vi "Remove Constant Current.vi"(0 "Device Name":string="Dev4", 1 "Device/Ports/Lines":string="Dev1/port0/line1,Dev1/port0/line5,Dev1/port0/line13,Dev1/port0/line15,Dev1/port0/line31,Dev1/port0/line30,Dev1/port0/line29,Dev1/port0/line26,Dev1/port0/line25,Dev1/port0/line24,Dev1/port0/line23,Dev1/port0/line22,Dev1/port0/line21,Dev1/port0/line20,Dev1/port0/line19,Dev1/port0/line18,Dev1/port0/line17\n", 3 "error in":errorcluster) -> (10 "error out":errorcluster)   [LabVIEW 2015]
panel:
  # "True means close relay"
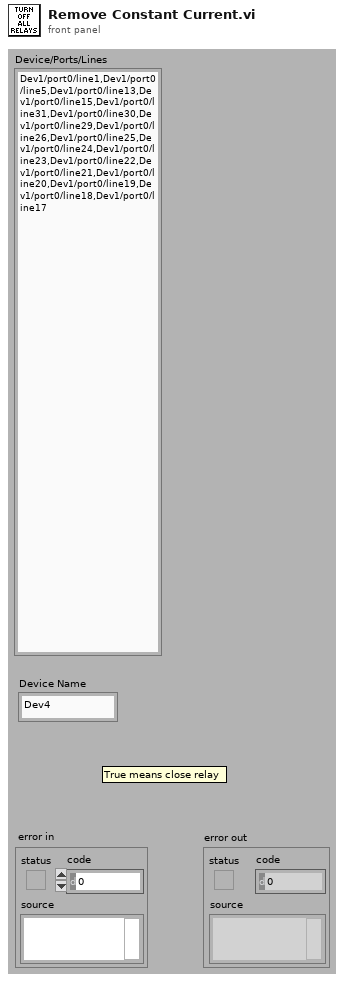
[diagram p1: front panel]
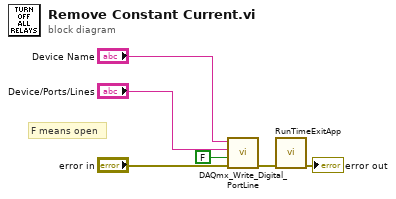
[diagram p0: block diagram]
diagram:
  # "F means open"
  n1 = call "DAQmx_Write_Digital_PortLine.vi"("Device/Ports/Lines"="Device Name", 1:"Device/Ports/Lines", "Boolean"=FALSE, "error in"="error in") -> ("error out"=w5:errorcluster)  [unwired: 5 in, 1 out]
  n2 = call "RunTimeExitApp.vi"("error in (no error)"=w5) -> ("error out"=→"error out":errorcluster)  [unwired: 10 in]
